vi "main.vi"() -> ()   [LabVIEW 2018]
panel:
  in  "connect button":bool
  out "connected?":bool
  in  "V11":bool
  in  "V10":bool
  in  "V9":bool
  in  "V8":bool
  in  "V7":bool
  in  "V6":bool
  in  "V5":bool
  in  "V4":bool
  in  "V3":bool
  in  "V2":bool
  in  "V1":bool
  in  "error in (no error)":errorcluster
  in  "VISA resource name":refnum<visa-resource-name>="COM4"
  # "SwitchBoxConrad"
  # "build 20181102, Ronny Friedrich"
  # "Valve Control"
  # "Card 1"
  # "Card 2"
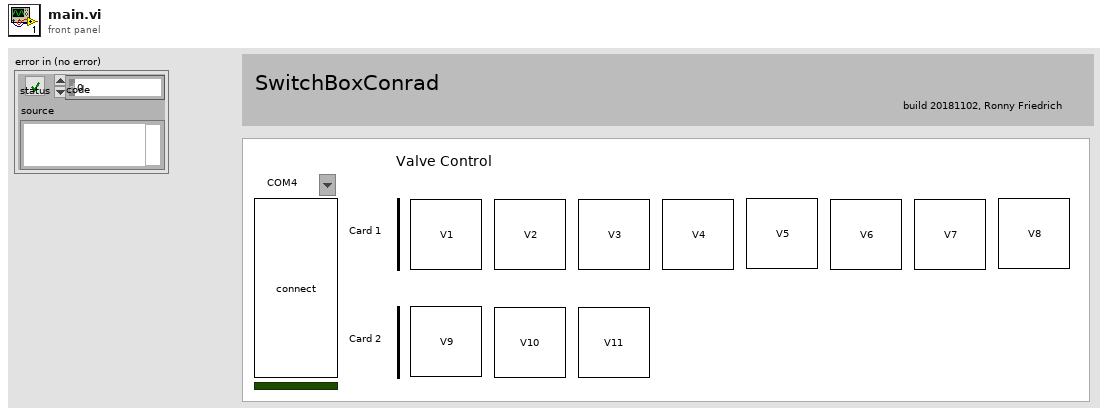
[diagram p1: front panel]
types:
  T1 = enum8{"Enabled", "Disabled", "Disabled and Grayed Out"}
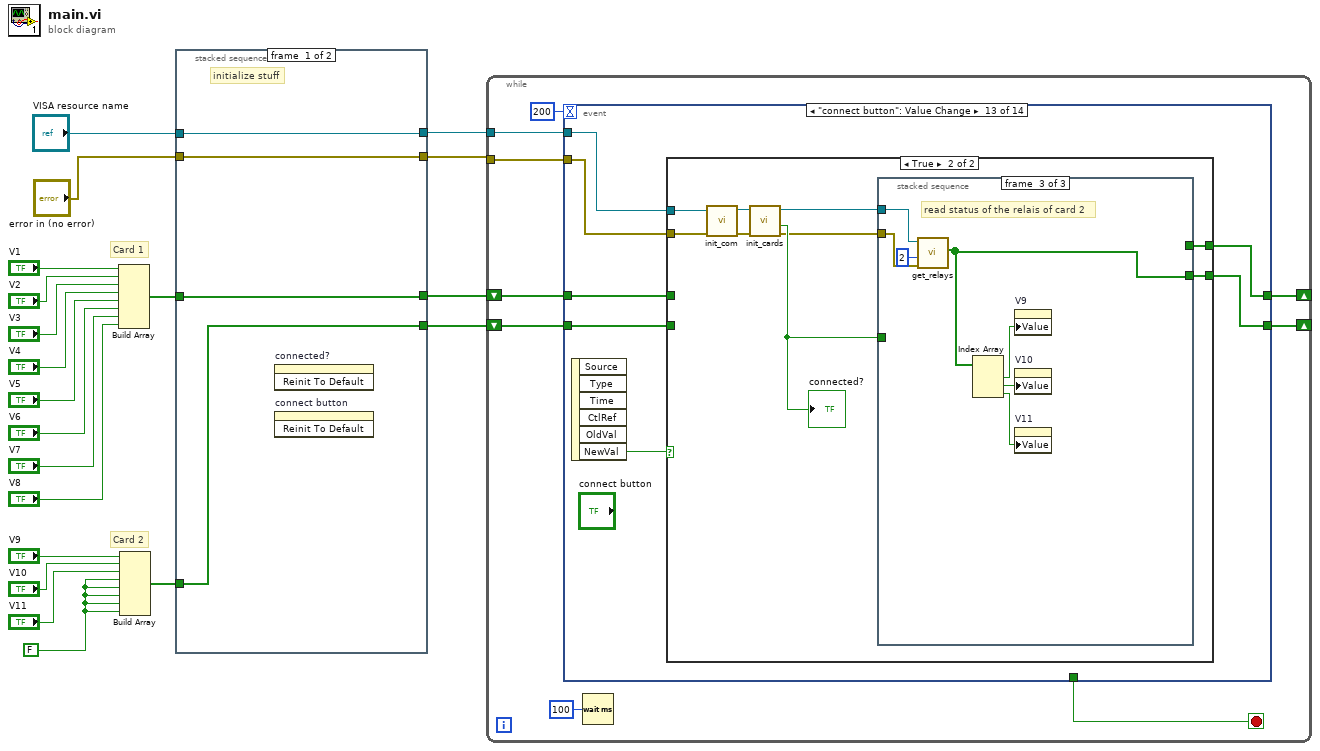
[diagram p0: block diagram]
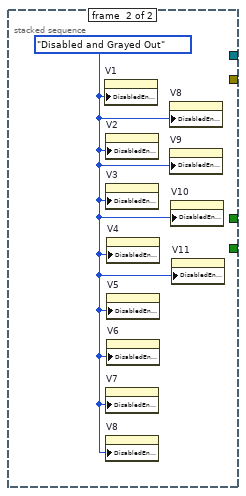
[diagram p2: hidden frame]
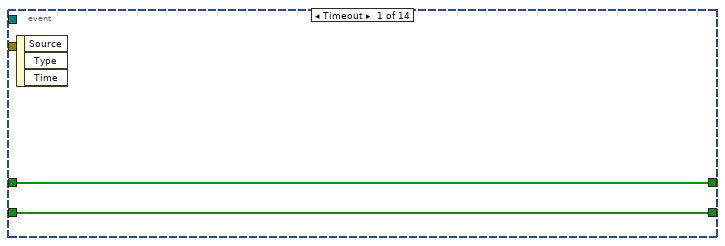
[diagram p3: hidden frame]
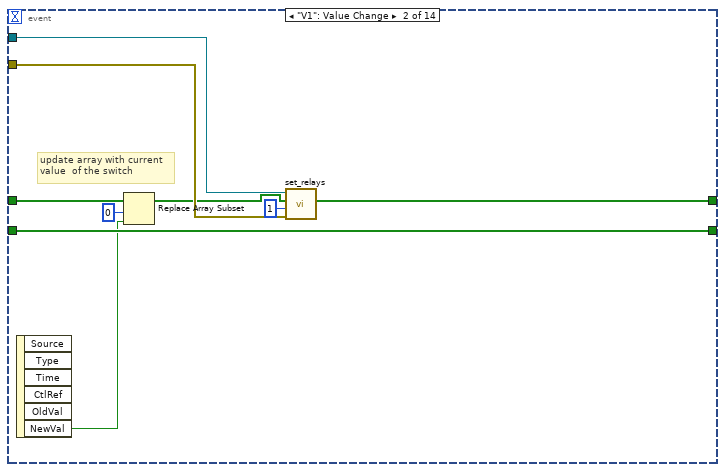
[diagram p4: hidden frame]
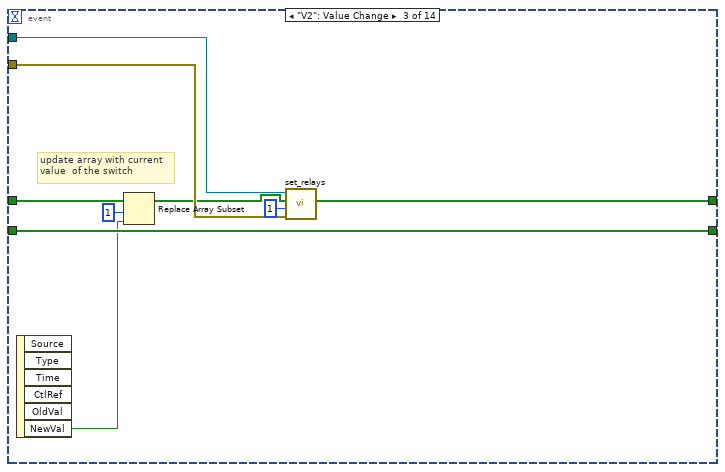
[diagram p5: hidden frame]
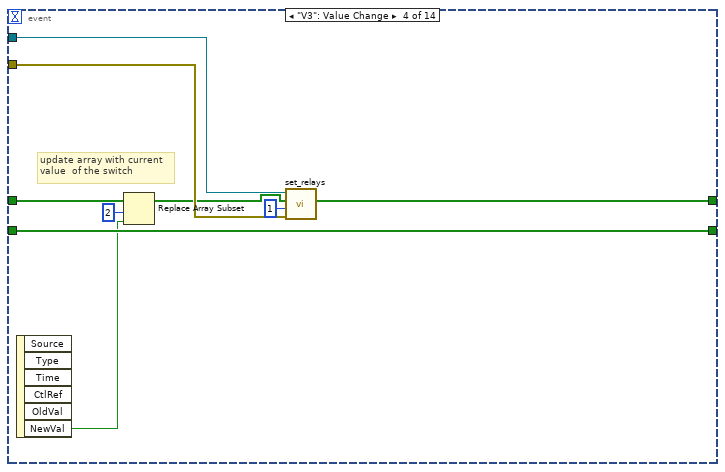
[diagram p6: hidden frame]
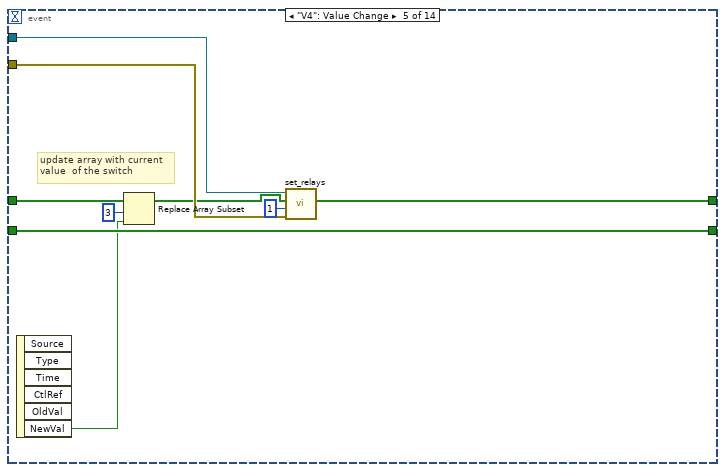
[diagram p7: hidden frame]
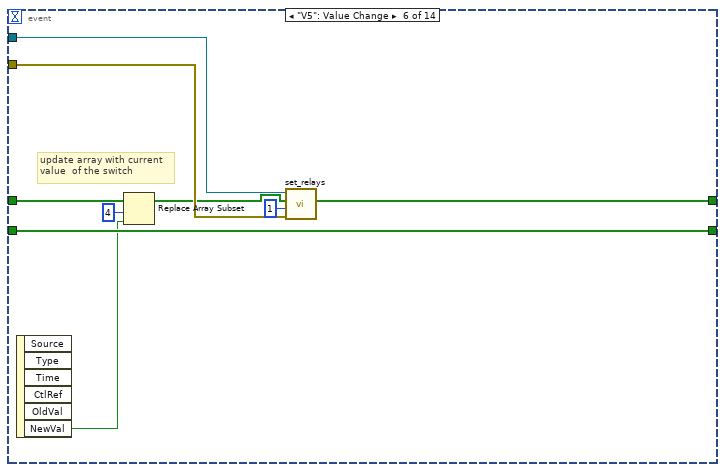
[diagram p8: hidden frame]
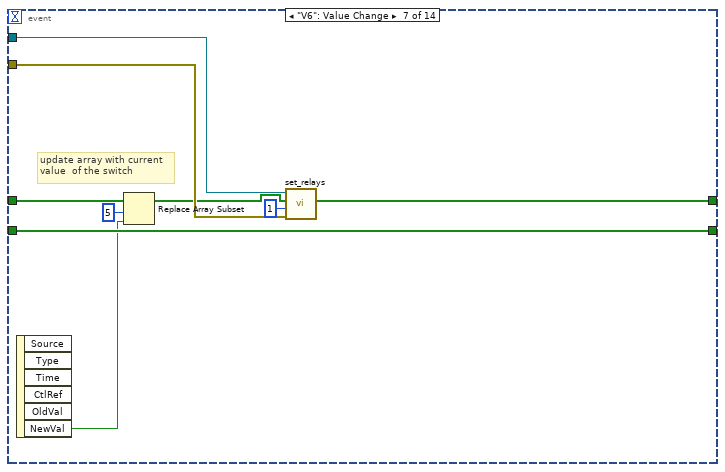
[diagram p9: hidden frame]
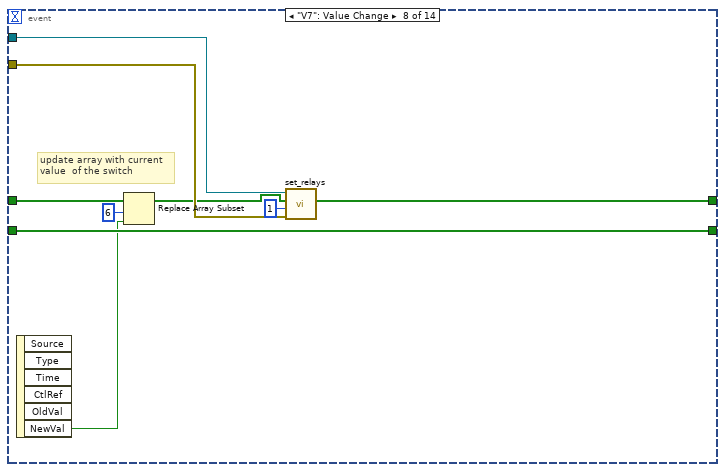
[diagram p10: hidden frame]
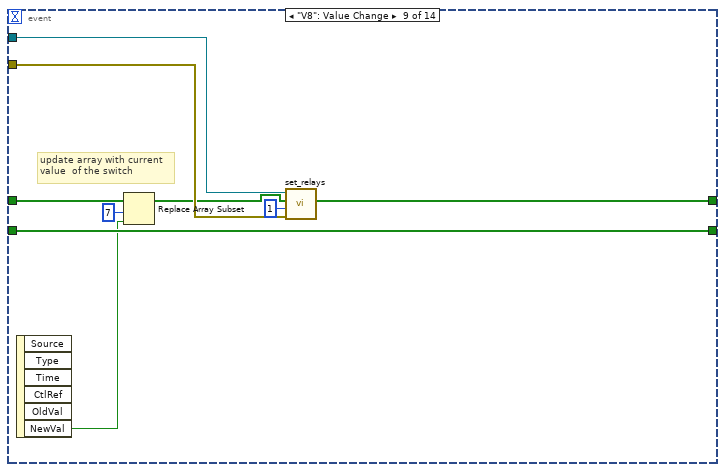
[diagram p11: hidden frame]
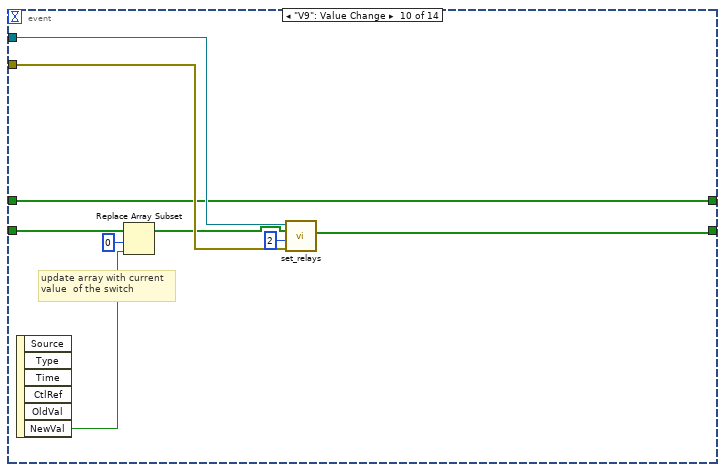
[diagram p12: hidden frame]
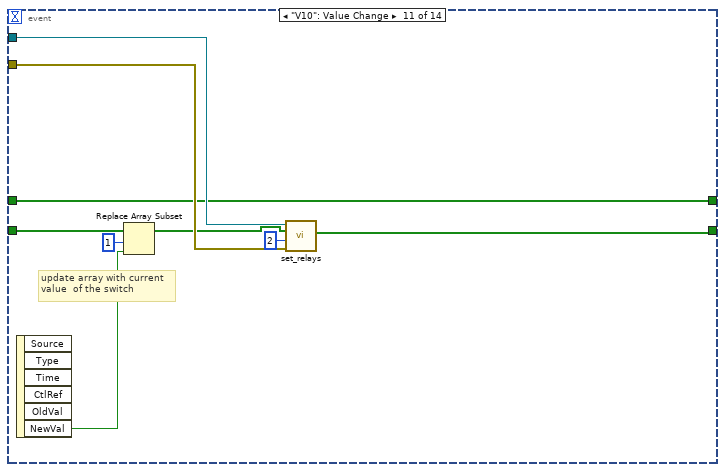
[diagram p13: hidden frame]
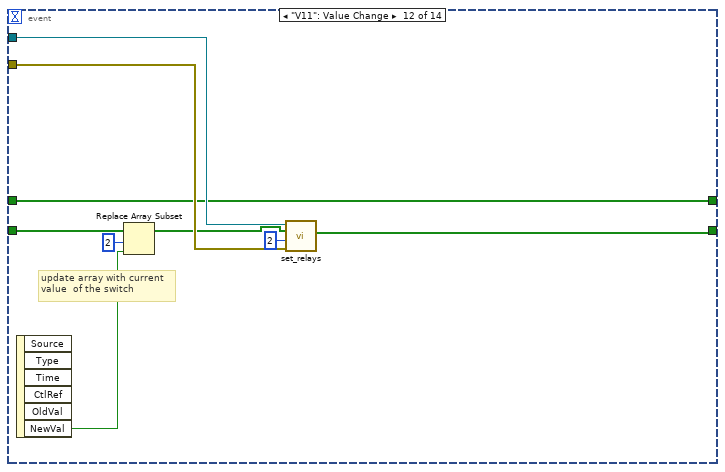
[diagram p14: hidden frame]
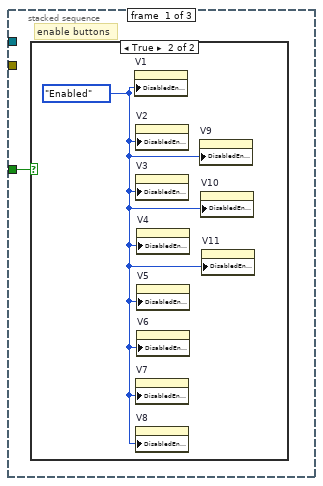
[diagram p16: hidden frame]
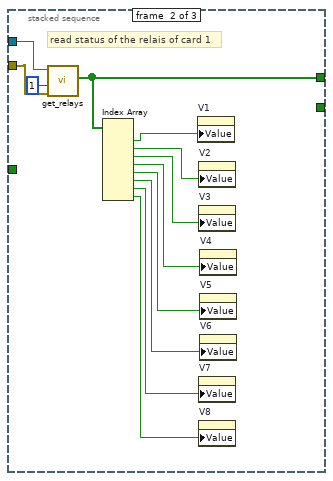
[diagram p18: hidden frame]
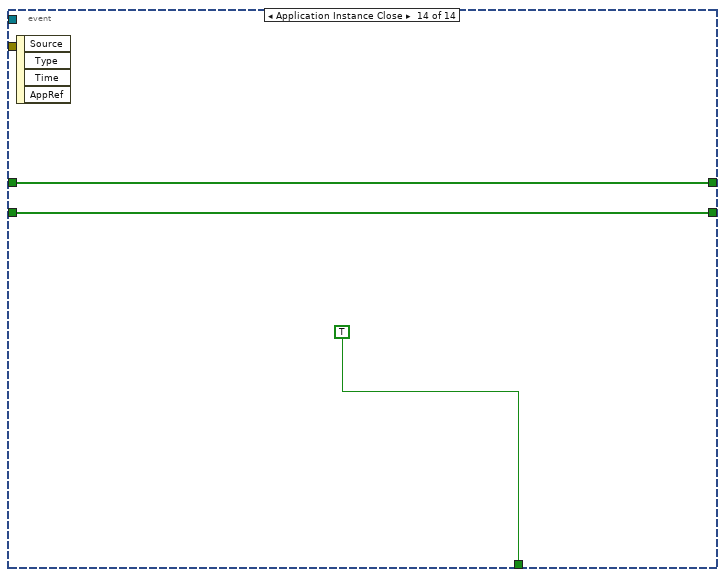
[diagram p19: hidden frame]
diagram:
  w3 = FALSE
  # "Card 2"
  # "Card 1"
  n1 = Build Array("V1", "V2", "V3", "V4", "V5", "V6", "V7", "V8") -> (w10:bool[])
  n2 = Build Array("V9", "V10", "V11", w3, w3, w3, w3, w3) -> (w6:bool[])
  n3 = stacked-sequence {
    tunnel: "VISA resource name" -> [w22 _]
    tunnel: [w21 _] -> w1
    tunnel: [w22 _] -> w2
    tunnel: "error in (no error)" -> [w21 _]
    tunnel: w10 -> [w24 _]
    tunnel: [w24 _] -> w5
    tunnel: w6 -> [w23 _]
    tunnel: [w23 _] -> w4
    frame #0 {
      # "initialize stuff"
      n4 = invoke on="connected?" class="Bool (strict)" method="Reinit To Default"() -> ()  [unwired: 3 in, 3 out]
      n5 = invoke on="connect button" class="Bool (strict)" method="Reinit To Default"() -> ()  [unwired: 3 in, 3 out]
    }
    frame #1 {
      w25 = T1."Disabled and Grayed Out" ("Disabled")
      n6 = property on="V1" class="Bool (strict)"("DisabledEnum"=w25) -> ()  [unwired: 2 in, 2 out]
      n7 = property on="V2" class="Bool (strict)"("DisabledEnum"=w25) -> ()  [unwired: 2 in, 2 out]
      n8 = property on="V3" class="Bool (strict)"("DisabledEnum"=w25) -> ()  [unwired: 2 in, 2 out]
      n9 = property on="V7" class="Bool (strict)"("DisabledEnum"=w25) -> ()  [unwired: 2 in, 2 out]
      n10 = property on="V8" class="Bool (strict)"("DisabledEnum"=w25) -> ()  [unwired: 2 in, 2 out]
      n11 = property on="V4" class="Bool (strict)"("DisabledEnum"=w25) -> ()  [unwired: 2 in, 2 out]
      n12 = property on="V5" class="Bool (strict)"("DisabledEnum"=w25) -> ()  [unwired: 2 in, 2 out]
      n13 = property on="V6" class="Bool (strict)"("DisabledEnum"=w25) -> ()  [unwired: 2 in, 2 out]
      n14 = property on="V8" class="Bool (strict)"("DisabledEnum"=w25) -> ()  [unwired: 2 in, 2 out]
      n15 = property on="V9" class="Bool (strict)"("DisabledEnum"=w25) -> ()  [unwired: 2 in, 2 out]
      n16 = property on="V10" class="Bool (strict)"("DisabledEnum"=w25) -> ()  [unwired: 2 in, 2 out]
      n17 = property on="V11" class="Bool (strict)"("DisabledEnum"=w25) -> ()  [unwired: 2 in, 2 out]
    }
  }
  n18 = while {
    tunnel: w2 -> [w29]
    tunnel: w1 -> [w28]
    shift-right: [w27] -> _
    shift-left: w5 -> [w31]
    shift-right: [w26] -> _
    shift-left: w4 -> [w30]
    stop <- w32 stop-if-true
    n19 = event shown="[12] \"connect button\": Value Change" {
      selector: _ -> [_ _ _ _ _ _ _ _ _ _ _ _ _ _]
      dyn-events: _ -> [_ _ _ _ _ _ _ _ _ _ _ _ _ _]
      timeout: 200 -> [_ _ _ _ _ _ _ _ _ _ _ _ _ _]
      tunnel: [_ _ _ _ _ _ _ _ _ _ _ _ _ TRUE] -> w32
      tunnel: w31 -> [w36 w40 w49 w58 w67 w76 w85 w94 w103 w109 w118 w127 w139 w176]
      tunnel: w30 -> [w35 w43 w52 w61 w70 w79 w88 w97 w106 w112 w121 w130 w138 w175]
      tunnel: w29 -> [_ w44 w53 w62 w71 w80 w89 w98 w107 w116 w125 w134 w140 _]
      tunnel: w28 -> [_ w45 w54 w63 w72 w81 w90 w99 w108 w117 w126 w135 w141 _]
      tunnel: [w36 w42 w51 w60 w69 w78 w87 w96 w105 w109 w118 w127 w137 w176] -> w27
      tunnel: [w35 w43 w52 w61 w70 w79 w88 w97 w106 w110 w119 w128 w136 w175] -> w26
      event Timeout {
        n20 = event-data() -> ()  [unwired: 1 in, 3 out]
      }
      event "V1": Value Change {
        # "update array with current\nvalue  of the switch"
        n21 = event-data() -> ("NewVal"=w38:bool)  [unwired: 1 in, 5 out]
        n22 = Replace Array Subset(array=w40, new element=w38, index=0) -> (w37:bool[])
        n23 = call "set_relays.vi"("error in (no error)"=w45, "card address"=u8 1, "boolian array in"=w37, "VISA Refnum in"=w44) -> ("boolian array out"=w42:bool[])  [unwired: 4 in, 3 out]
      }
      event "V2": Value Change {
        # "update array with current\nvalue  of the switch"
        n24 = event-data() -> ("NewVal"=w47:bool)  [unwired: 1 in, 5 out]
        n25 = Replace Array Subset(array=w49, new element=w47, index=1) -> (w46:bool[])
        n26 = call "set_relays.vi"("error in (no error)"=w54, "card address"=u8 1, "boolian array in"=w46, "VISA Refnum in"=w53) -> ("boolian array out"=w51:bool[])  [unwired: 4 in, 3 out]
      }
      event "V3": Value Change {
        # "update array with current\nvalue  of the switch"
        n27 = event-data() -> ("NewVal"=w56:bool)  [unwired: 1 in, 5 out]
        n28 = Replace Array Subset(array=w58, new element=w56, index=2) -> (w55:bool[])
        n29 = call "set_relays.vi"("error in (no error)"=w63, "card address"=u8 1, "boolian array in"=w55, "VISA Refnum in"=w62) -> ("boolian array out"=w60:bool[])  [unwired: 4 in, 3 out]
      }
      event "V4": Value Change {
        # "update array with current\nvalue  of the switch"
        n30 = event-data() -> ("NewVal"=w65:bool)  [unwired: 1 in, 5 out]
        n31 = Replace Array Subset(array=w67, new element=w65, index=3) -> (w64:bool[])
        n32 = call "set_relays.vi"("error in (no error)"=w72, "card address"=u8 1, "boolian array in"=w64, "VISA Refnum in"=w71) -> ("boolian array out"=w69:bool[])  [unwired: 4 in, 3 out]
      }
      event "V5": Value Change {
        # "update array with current\nvalue  of the switch"
        n33 = event-data() -> ("NewVal"=w74:bool)  [unwired: 1 in, 5 out]
        n34 = Replace Array Subset(array=w76, new element=w74, index=4) -> (w73:bool[])
        n35 = call "set_relays.vi"("error in (no error)"=w81, "card address"=u8 1, "boolian array in"=w73, "VISA Refnum in"=w80) -> ("boolian array out"=w78:bool[])  [unwired: 4 in, 3 out]
      }
      event "V6": Value Change {
        # "update array with current\nvalue  of the switch"
        n36 = event-data() -> ("NewVal"=w83:bool)  [unwired: 1 in, 5 out]
        n37 = Replace Array Subset(array=w85, new element=w83, index=5) -> (w82:bool[])
        n38 = call "set_relays.vi"("error in (no error)"=w90, "card address"=u8 1, "boolian array in"=w82, "VISA Refnum in"=w89) -> ("boolian array out"=w87:bool[])  [unwired: 4 in, 3 out]
      }
      event "V7": Value Change {
        # "update array with current\nvalue  of the switch"
        n39 = event-data() -> ("NewVal"=w92:bool)  [unwired: 1 in, 5 out]
        n40 = Replace Array Subset(array=w94, new element=w92, index=6) -> (w91:bool[])
        n41 = call "set_relays.vi"("error in (no error)"=w99, "card address"=u8 1, "boolian array in"=w91, "VISA Refnum in"=w98) -> ("boolian array out"=w96:bool[])  [unwired: 4 in, 3 out]
      }
      event "V8": Value Change {
        # "update array with current\nvalue  of the switch"
        n42 = event-data() -> ("NewVal"=w101:bool)  [unwired: 1 in, 5 out]
        n43 = Replace Array Subset(array=w103, new element=w101, index=7) -> (w100:bool[])
        n44 = call "set_relays.vi"("error in (no error)"=w108, "card address"=u8 1, "boolian array in"=w100, "VISA Refnum in"=w107) -> ("boolian array out"=w105:bool[])  [unwired: 4 in, 3 out]
      }
      event "V9": Value Change {
        # "update array with current\nvalue  of the switch"
        n45 = event-data() -> ("NewVal"=w113:bool)  [unwired: 1 in, 5 out]
        n46 = Replace Array Subset(array=w112, new element=w113, index=0) -> (w111:bool[])
        n47 = call "set_relays.vi"("error in (no error)"=w117, "card address"=u8 2, "boolian array in"=w111, "VISA Refnum in"=w116) -> ("boolian array out"=w110:bool[])  [unwired: 4 in, 3 out]
      }
      event "V10": Value Change {
        # "update array with current\nvalue  of the switch"
        n48 = event-data() -> ("NewVal"=w122:bool)  [unwired: 1 in, 5 out]
        n49 = Replace Array Subset(array=w121, new element=w122, index=1) -> (w120:bool[])
        n50 = call "set_relays.vi"("error in (no error)"=w126, "card address"=u8 2, "boolian array in"=w120, "VISA Refnum in"=w125) -> ("boolian array out"=w119:bool[])  [unwired: 4 in, 3 out]
      }
      event "V11": Value Change {
        # "update array with current\nvalue  of the switch"
        n51 = event-data() -> ("NewVal"=w131:bool)  [unwired: 1 in, 5 out]
        n52 = Replace Array Subset(array=w130, new element=w131, index=2) -> (w129:bool[])
        n53 = call "set_relays.vi"("error in (no error)"=w135, "card address"=u8 2, "boolian array in"=w129, "VISA Refnum in"=w134) -> ("boolian array out"=w128:bool[])  [unwired: 4 in, 3 out]
      }
      event "connect button": Value Change {
        n54 = event-data() -> ("NewVal"=w142:bool)  [unwired: 1 in, 5 out]
        n55 = case shown="True" w142 {
          tunnel: w141 -> [_ w151]
          tunnel: w140 -> [_ w150]
          tunnel: w139 -> [w144 _]
          tunnel: w138 -> [w143 _]
          tunnel: [w144 w146] -> w137
          tunnel: [w143 w145] -> w136
          frame False {
          }
          frame True {
            n56 = call "init_com.vi"("error in (no error)"=w151, "VISA Refnum in"=w150) -> ("error out"=w152:errorcluster, "VISA Refnum out"=w153:refnum<visa-resource-name>)  [unwired: 8 in]
            n57 = call "init_cards.vi"("error in (no error)"=w152, "VISA Refnum in"=w153) -> ("error out"=w148:errorcluster, "init ok?"=w149:bool, "VISA Refnum out"=w147:refnum<visa-resource-name>)  [unwired: 6 in, 1 out]
            "connected?" <- w149
            n58 = stacked-sequence {
              tunnel: w149 -> [w154 _ _]
              tunnel: w148 -> [_ w166 w173]
              tunnel: w147 -> [_ w167 w174]
              tunnel: [_ w156 _] -> w146
              tunnel: [_ _ w168] -> w145
              frame #0 {
                # "enable buttons"
                n59 = case shown="True" w154 {
                  frame False {
                  }
                  frame True {
                    w155 = T1."Enabled" ("Disabled")
                    n60 = property on="V1" class="Bool (strict)"("DisabledEnum"=w155) -> ()  [unwired: 2 in, 2 out]
                    n61 = property on="V2" class="Bool (strict)"("DisabledEnum"=w155) -> ()  [unwired: 2 in, 2 out]
                    n62 = property on="V3" class="Bool (strict)"("DisabledEnum"=w155) -> ()  [unwired: 2 in, 2 out]
                    n63 = property on="V7" class="Bool (strict)"("DisabledEnum"=w155) -> ()  [unwired: 2 in, 2 out]
                    n64 = property on="V8" class="Bool (strict)"("DisabledEnum"=w155) -> ()  [unwired: 2 in, 2 out]
                    n65 = property on="V4" class="Bool (strict)"("DisabledEnum"=w155) -> ()  [unwired: 2 in, 2 out]
                    n66 = property on="V5" class="Bool (strict)"("DisabledEnum"=w155) -> ()  [unwired: 2 in, 2 out]
                    n67 = property on="V6" class="Bool (strict)"("DisabledEnum"=w155) -> ()  [unwired: 2 in, 2 out]
                    n68 = property on="V9" class="Bool (strict)"("DisabledEnum"=w155) -> ()  [unwired: 2 in, 2 out]
                    n69 = property on="V10" class="Bool (strict)"("DisabledEnum"=w155) -> ()  [unwired: 2 in, 2 out]
                    n70 = property on="V11" class="Bool (strict)"("DisabledEnum"=w155) -> ()  [unwired: 2 in, 2 out]
                  }
                }
              }
              frame #1 {
                # "read status of the relais of card 1"
                n71 = call "get_relays.vi"("error in (no error)"=w166, "card address"=u8 1, "VISA Refnum in"=w167) -> ("boolian array out"=w156:bool[])  [unwired: 5 in, 3 out]
                n72 = Index Array(array=w156) -> (element #1=w165:bool, element #2=w164:bool, element #3=w163:bool, element #4=w162:bool, element #5=w161:bool, element #6=w160:bool, element #7=w159:bool, element #8=w158:bool)  [unwired: 8 in]
                n73 = property on="V1" class="Bool (strict)"("Value"=w165) -> ()  [unwired: 2 in, 2 out]
                n74 = property on="V2" class="Bool (strict)"("Value"=w164) -> ()  [unwired: 2 in, 2 out]
                n75 = property on="V3" class="Bool (strict)"("Value"=w163) -> ()  [unwired: 2 in, 2 out]
                n76 = property on="V7" class="Bool (strict)"("Value"=w159) -> ()  [unwired: 2 in, 2 out]
                n77 = property on="V8" class="Bool (strict)"("Value"=w158) -> ()  [unwired: 2 in, 2 out]
                n78 = property on="V4" class="Bool (strict)"("Value"=w162) -> ()  [unwired: 2 in, 2 out]
                n79 = property on="V5" class="Bool (strict)"("Value"=w161) -> ()  [unwired: 2 in, 2 out]
                n80 = property on="V6" class="Bool (strict)"("Value"=w160) -> ()  [unwired: 2 in, 2 out]
              }
              frame #2 {
                # "read status of the relais of card 2"
                n81 = call "get_relays.vi"("error in (no error)"=w173, "card address"=u8 2, "VISA Refnum in"=w174) -> ("boolian array out"=w168:bool[])  [unwired: 5 in, 3 out]
                n82 = Index Array(array=w168) -> (element #1=w171:bool, element #2=w170:bool, element #3=w169:bool)  [unwired: 3 in]
                n83 = property on="V9" class="Bool (strict)"("Value"=w171) -> ()  [unwired: 2 in, 2 out]
                n84 = property on="V10" class="Bool (strict)"("Value"=w170) -> ()  [unwired: 2 in, 2 out]
                n85 = property on="V11" class="Bool (strict)"("Value"=w169) -> ()  [unwired: 2 in, 2 out]
              }
            }
          }
        }
      }
      event Application Instance Close {
        n86 = event-data() -> ()  [unwired: 1 in, 4 out]
      }
    }
    n87 = Wait (ms)(milliseconds to wait=u32 100) -> ()  [unwired: 1 out]
  }
